vi "error-199203001.vi"(9 "数据":variant, 10 "字符串":string, 11 "VI输入":refnum<vi>) -> (0 "错误输出":errorcluster)   [LabVIEW 2014]
uses:
  R-Error.vi
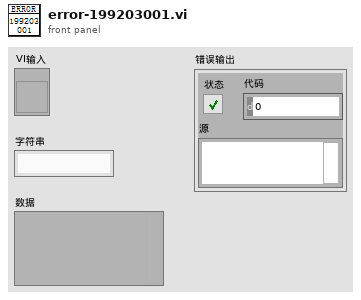
[diagram p1: front panel]
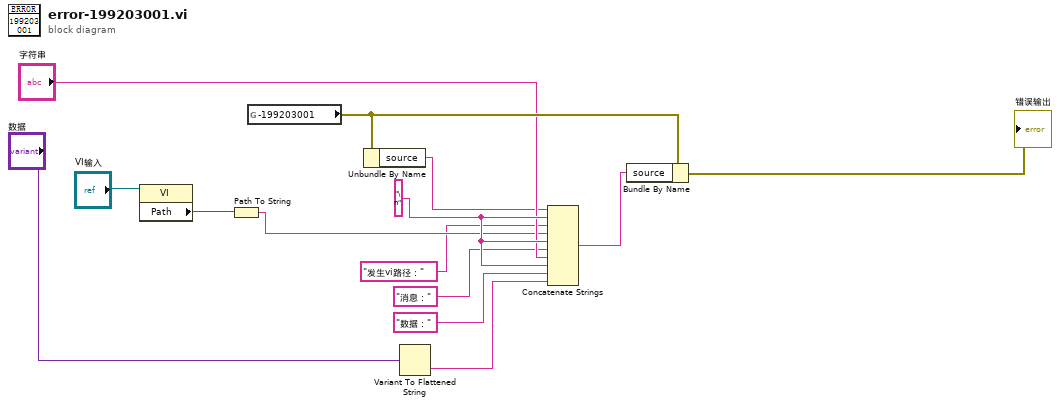
[diagram p0: block diagram]
diagram:
  w8 = "\n" ("字符串")
  n1 = property class="VI"(reference="VI输入") -> ("Path"=w4:path)  [unwired: 1 in, 2 out]
  n2 = Path To String(path=w4) -> (string=w5:string)
  n3 = global read "R-Error.vi" "-199203001"() -> (w12:errorcluster)
  n4 = Unbundle By Name(w12) -> ("source"=w2:string)
  n5 = Variant To Flattened String(Variant="数据") -> (data string=w11:string)  [unwired: 1 out]
  n6 = Concatenate Strings(w2, w8, "发生vi路径：" ("字符串"), w5, w8, "消息：" ("字符串"), "字符串", w8, "数据：" ("字符串"), w11) -> (w13:string)
  n7 = Bundle By Name(cluster=w12, "source"=w13) -> (→"错误输出":errorcluster)
